vi "5782_input_test.vi"() -> ()   [LabVIEW 2013]
uses:
  FPGA/DataMode.ctl
  <vilib>/Platform/TimedLoop/XDataNode/timing_clust.ctl
  <vilib>/Platform/TimedLoop/XDataNode/nitl_modes.ctl
  <vilib>/Platform/TimedLoop/XDataNode/wakeup.ctl
  <vilib>/rvi/Emulation/niFpgaSctlEmulationGetInTimedLoop.vi
  <vilib>/rvi/Emulation/niFpgaEmulationReportErrorSimple.vi
  <vilib>/rvi/Emulation/niFpgaGetClockAttributes.vi
  <vilib>/rvi/Emulation/niFpgaCriticalErrorInLSC.vi
  <vilib>/rvi/interface/RandomDataEmulation/nirviRandomDataFPGAFIFO.vi
  <vilib>/rvi/interface/RandomDataEmulation/niFpgaRandomDataHandleErrors.vi
  <vilib>/rvi/eio/common/nirviEmuTemplateMethod_errors.vi
  <vilib>/rvi/FIFO/Fifo_Resource/nirvififoEmulationReadFpgaImpl.vi
  <vilib>/rvi/DataTransferAndStorage/Container/Common/niFpgaContainerGetUniqueNameForEmu.vi
  <vilib>/rvi/FIFO/Fifo_Resource/nirvififoEmulationWriteFpgaImpl.vi
  <vilib>/Platform/TimedLoop/XDataNode/XDataNode.xnode
  <vilib>/rvi/DataTransferAndStorage/Container/XNode/niFpgaContainer.xnode
  <vilib>/rvi/interface/RandomDataEmulation/nirviRandomDataFpgaReadWriteTemplate.vi
  <vilib>/eio/EIONode/EIONode.xnode
  <vilib>/rvi/FIFO/Fifo_Resource/nirvififoEmulationRead.vi
  <vilib>/rvi/FIFO/Fifo_Resource/nirvififoEmulationWrite.vi
  <vilib>/Platform/TimedLoop/XDataNode/XDNodeRunTimeDep.lvlib
panel:
  in  "downsample rate":u32=500
  in  "Trigger Acquisition":bool
  in  "Simulated phase 5782":fxp<+,64,64>[](array[numeric])=[0.0, 0.0]
  in  "Mode":T1
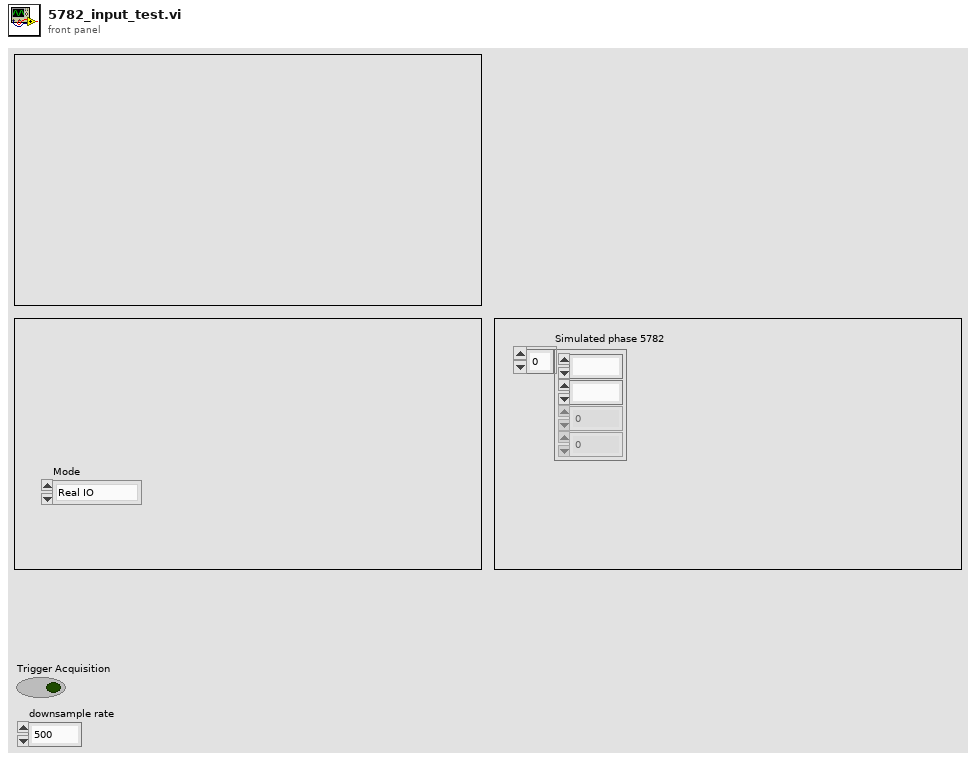
[diagram p1: front panel]
types:
  T1 = typedef "DataMode.ctl" = enum16{"Real IO", "Simulated"}
  T2 = typedef "XDNodeRunTimeDep.lvlib/timing_clust.ctl" = cluster{"Expected End [f-1]":u64, "Actual End [f-1]":u64, "Finished Late? [f-1]":bool, "Expected End [i-1]":u64, "Actual End [i-1]":u64, "Finished Late? [i-1]":bool, "Expected Start [i]":u64, "Actual Start [i]":u64, "Expected Start [f]":u64, "Actual Start [f]":u64, "Source Name":string, "Structure Name":string, "Period":i64, "Deadline":i64, "Offset":i64, "Start":i64, "Priority":i32, "Timeout":i32, "Mode":T3, "Wakeup Reason":T4, "Error":errorcluster, "Source Type":string, "Secondary Source Type":string, "Global End Time":u64, "Global Start Time":u64, "Frame Duration":u64, "Iteration Duration":u64, "Assigned CPU":i32, "I/O Scan Engine Mode":u32}
  T3 = typedef "XDNodeRunTimeDep.lvlib/nitl_modes.ctl" = enum32{"No Change", "Process missed periods, maintain original phase", "Discard missed periods, maintain original phase", "Process missed periods, ignore original phase", "Discard missed periods, ignore original phase"}
  T4 = typedef "XDNodeRunTimeDep.lvlib/wakeup.ctl" = enum32{"Normal", "Aborted", "Asynchronous wakeup", "Timing source error", "Timed loop error", "Timeout"}
  T5 = typedef "I16 array size 2.ctl" = i16[]
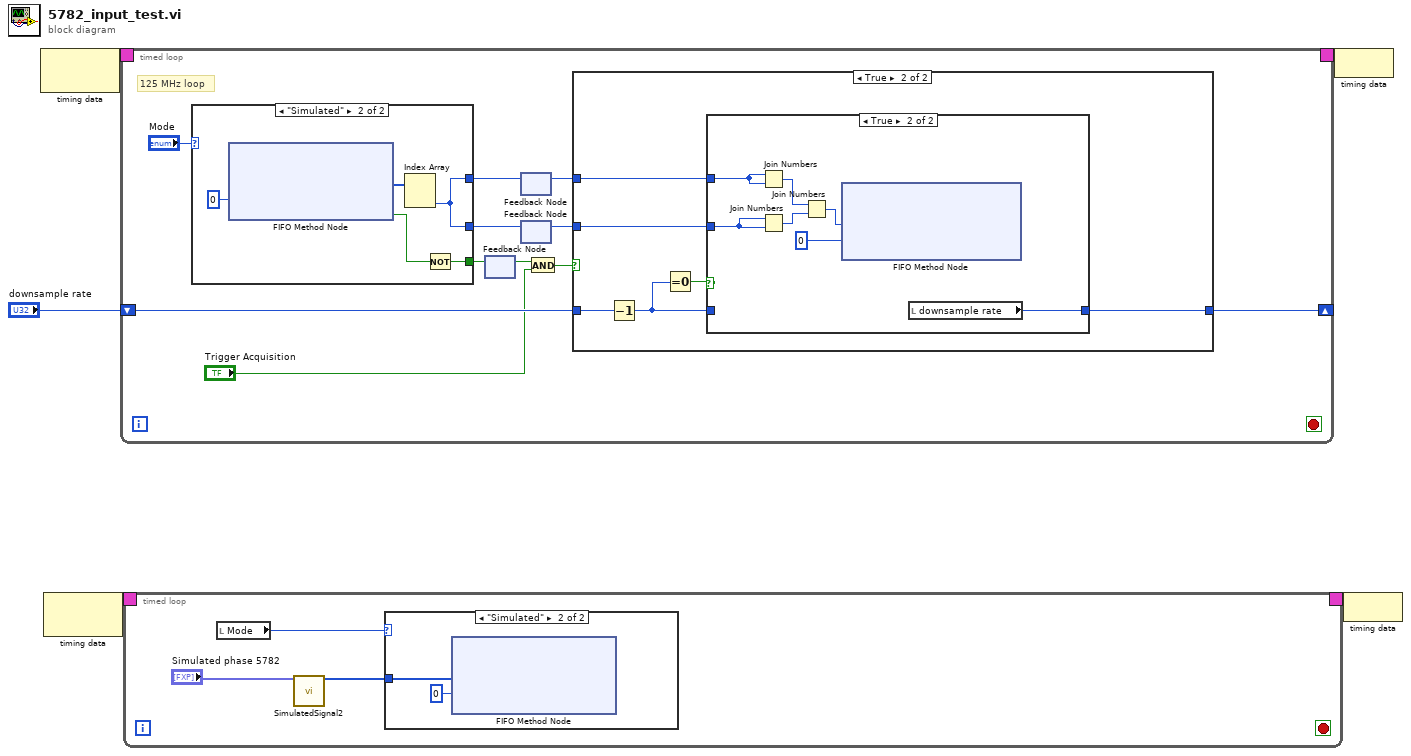
[diagram p0: block diagram]
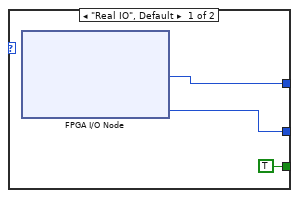
[diagram p4: hidden frame]
diagram:
  n1 = node-c288() -> (w3:T2)  [unwired: 1 in]
  n2 = node-c288() -> (w5:T2)  [unwired: 1 in]
  n3 = timed-loop {
    timing: w3 -> [_]
    timing-out: [_] -> w2
    shift-right: [w9] -> _
    shift-left: "downsample rate" -> [w10]
    stop <- _ stop-if-true
    # "125 MHz loop"
    n4 = case shown="\"Simulated\"" "Mode" {
      tunnel: [w34 w37] -> w15
      tunnel: [w33 w37] -> w12
      tunnel: [TRUE w35] -> w11
      frame "Real IO", Default {
        n5 = xnode "FPGA I/O Node"() -> ("IO Module\\AI 0 N"=w34:i16, "IO Module\\AI 1 N"=w33:i16)  [unwired: 4 in, 6 out]
      }
      frame "Simulated" {
        n6 = xnode ("FIFO Method Node")("Timeout"=0) -> ("Element"=w38:i16[], "Timed Out?"=w36:bool)  [unwired: 1 in, 1 out]
        n7 = Index Array(array=w38) -> (element #2=w37:i16)  [unwired: 2 in, 1 out]
        n8 = Not(x=w36) -> (.not. x?=w35:bool)
      }
    }
    n9 = feedback #1() -> (w8:bool)  [unwired: 1 in]
    n10 = feedback-in #1(w11) -> ()
    n11 = feedback #2() -> (w14:i16)  [unwired: 1 in]
    n12 = feedback-in #2(w15) -> ()
    n13 = feedback #3() -> (w13:i16)  [unwired: 1 in]
    n14 = feedback-in #3(w12) -> ()
    n15 = And(x=w8, y="Trigger Acquisition") -> (x .and. y?=w7:bool)
    n16 = case shown="True" w7 {
      tunnel: w14 -> [_ w19]
      tunnel: w13 -> [_ w18]
      tunnel: w10 -> [w17 w23]
      tunnel: [w17 w21] -> w9
      frame False {
      }
      frame True {
        n17 = Decrement(x=w23) -> (x-1=w20:u32)
        n18 = Equal To 0?(x=w20) -> (x = 0?=w22:bool)
        n19 = case shown="True" w22 {
          tunnel: [w24 w31] -> w21
          tunnel: w20 -> [w24 _]
          tunnel: w19 -> [_ w27]
          tunnel: w18 -> [_ w26]
          frame False {
          }
          frame True {
            n20 = Join Numbers(hi=w27, lo=w27) -> ((hi.lo)=w29:u32)
            n21 = Join Numbers(hi=w26, lo=w26) -> ((hi.lo)=w28:u32)
            n22 = Join Numbers(hi=w29, lo=w28) -> ((hi.lo)=w25:u64)
            n23 = xnode ("FIFO Method Node")("Element"=w25, "Timeout"=0) -> ()  [unwired: 1 in, 2 out]
            n24 = local read "downsample rate"() -> (w31:u32)
          }
        }
      }
    }
  }
  n25 = timed-loop {
    timing: w5 -> [_]
    timing-out: [_] -> w4
    stop <- _ stop-if-true
    n26 = local read "Mode"() -> (w44:T1)
    n27 = call "SimulatedSignal2.vi"("Phase"="Simulated phase 5782") -> ("output"=w43:T5)  [unwired: 9 in, 1 out]
    n28 = case shown="\"Simulated\"" w44 {
      tunnel: w43 -> [_ w45]
      frame "Real IO", Default {
      }
      frame "Simulated" {
        n29 = xnode ("FIFO Method Node")("Element"=w45, "Timeout"=0) -> ()  [unwired: 1 in, 2 out]
      }
    }
  }
  n30 = node-c288(w2) -> ()
  n31 = node-c288(w4) -> ()
